vi "concatenate array.vi"(10 "reset":bool=TRUE, 11 "Array":cluster{"Array":dbl[], "Array":dbl[]}[](array[cluster])) -> (3 "appended array":cluster{"Array":dbl[], "Array":dbl[]}[](array[cluster]))   [LabVIEW 2021]
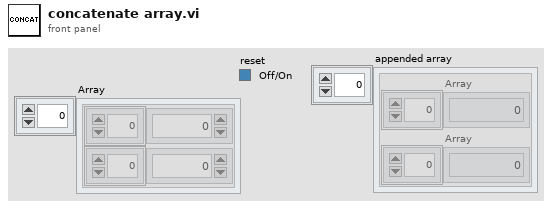
[diagram p1: front panel]
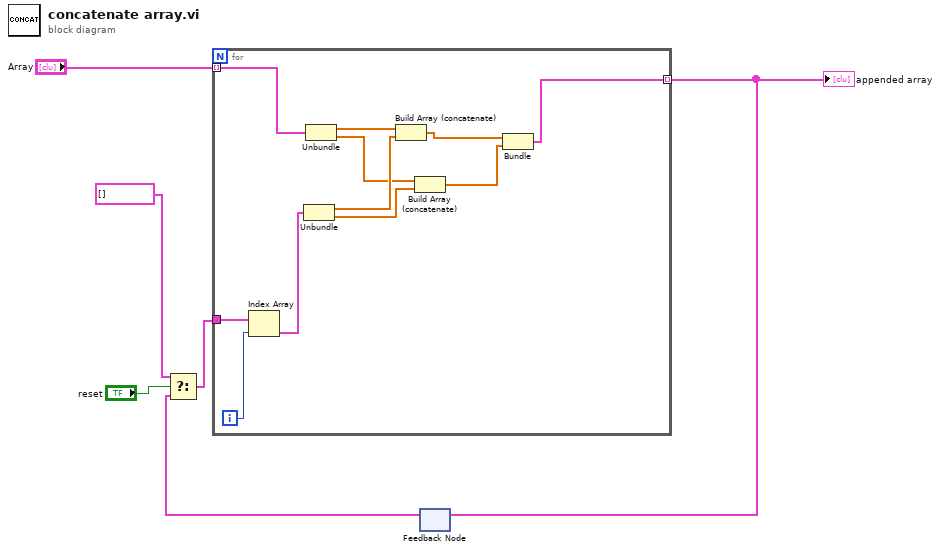
[diagram p0: block diagram]
diagram:
  n1 = feedback #1() -> (w2:cluster{dbl[], dbl[]}[])  [unwired: 1 in]
  n2 = Select(t=cluster{"Array":dbl[], "Array":dbl[]}[] [], s="reset", f=w2) -> (s? t:f=w3:cluster{"Array":dbl[], "Array":dbl[]}[])
  n3 = for {
    tunnel: [w10] -> w1 mode=indexing
    tunnel: "Array" -> [w17] mode=indexing
    tunnel: w3 -> [w9]
    i -> [w7]
    n4 = Index Array(array=w9, index=w7) -> (element=w8:cluster{"Array":dbl[], "Array":dbl[]})
    n5 = Unbundle(w8) -> ("Array"=w15:dbl[], "Array"=w13:dbl[])
    n6 = Unbundle(w17) -> ("Array"=w16:dbl[], "Array"=w14:dbl[])
    n7 = Build Array (concatenate)(w16, w15) -> (w12:dbl[])
    n8 = Build Array (concatenate)(w14, w13) -> (w11:dbl[])
    n9 = Bundle(w12, w11) -> (w10:cluster{dbl[], dbl[]})  [unwired: 1 in]
  }
  "appended array" <- w1
  n10 = feedback-in #1(w1) -> ()
